vi "test_ReentrantMeasurement_MultipleMeasureCalls_ExecuteInParallel.vi"(8 "error in":errorcluster) -> (0 "error out":errorcluster, 2 "result":string, 3 "pass":bool)   [LabVIEW 2021, in "MeasurementServerTests.lvlib" / "Measurement Service Tests.lvlib"]
uses:
  Measurement Service Tests.lvlib
  Runtime/Measurements/Helpers/TypeDefs/Measurement Server User Settings.ctl
  Runtime/Measurements/Helpers/TypeDefs/Stop Server User Event.ctl
  Runtime/Measurements/Helpers/TypeDefs/Measurement Service Version.ctl
  Continuous Counting Client/controls/Measurement Configuration.ctl
  f8b4024b-4f22-4a1f-8b12-3de1cba605e1.vi
  Runtime/Measurements/NI Measurement Plug-In SDK.lvlib
  Continuous Counting Client/Continuous Counting Client.lvlib
  Continuous Counting Measurement/Continuous Counting Measurement.lvclass
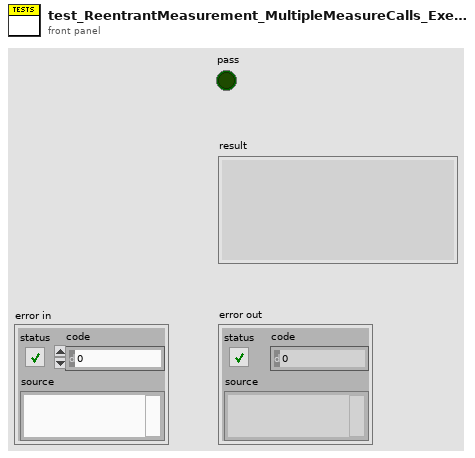
[diagram p1: front panel]
types:
  T1 = typedef "MeasurementServerTests.lvlib/Measurement Service Tests.lvlib/Continuous Counting Client.lvlib/Measurement Configuration.ctl" = cluster{"ms update interval":u32}
  T2 = typedef "NI Measurement Plug-In SDK.lvlib/Measurement Service Version.ctl" = enum16{"V1", "V2"}
  T3 = typedef "NI Measurement Plug-In SDK.lvlib/Measurement Server User Settings.ctl" = cluster{"stop server":T4, "measurement service versions":T2[]}
  T4 = typedef "NI Measurement Plug-In SDK.lvlib/Stop Server User Event.ctl" = refnum<user-event>
  T5 = typedef "grpc-lvsupport-release.lvlib/grpcId.ctl" = u64
  T6 = typedef "MeasurementServerTests.lvlib/Measurement Service Tests.lvlib/Continuous Counting Client.lvlib/Measurement Results.ctl" = cluster{"current count":i64}
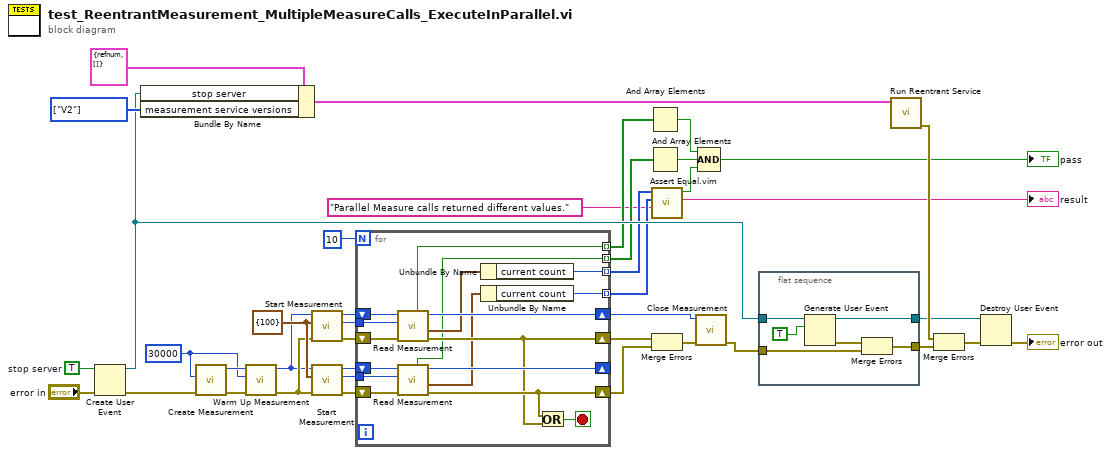
[diagram p0: block diagram]
diagram:
  w5 = 30000 ("ms timeout")
  w35 = T1 {"ms update interval"=100} ("measurement configuration")
  w38 = TRUE  # stop server
  w39 = T2[] [enum."V2"] items=["V1", "V2"] ("measurement service versions")
  n1 = Create User Event(user event datatype=w38, error in="error in") -> (user event=w22:refnum<user-event>, error out=w23:errorcluster)
  n2 = Bundle By Name(cluster=T3 {"stop server"=refnum, "measurement service versions"=[]} ("server settings"), "stop server"=w22, "measurement service versions"=w39) -> (w37:T3)
  n3 = call "Create Measurement.vi"("error in"=w23, "ms timeout"=w5) -> ("error out"=w9:errorcluster, "gRPCid out"=w7:T5)  [unwired: 8 in]
  n4 = call "Warm Up Measurement.vi"("error in"=w9, "timeout (ms)"=w5, "gRPC ID"=w7) -> ("error out"=w8:errorcluster, "gRPC ID out"=w6:T5)  [unwired: 6 in, 1 out]
  n5 = call "Start Measurement.vi"("error in"=w8, "measurement configuration"=w35, "gRPCid in"=w6) -> ("error out"=w32:errorcluster, "call id"=w33:T5, "gRPCid out"=w34:T5)  [unwired: 6 in]
  n6 = call "Start Measurement.vi"("error in"=w8, "measurement configuration"=w35, "gRPCid in"=w6) -> ("error out"=w30:errorcluster, "call id"=w29:T5, "gRPCid out"=w31:T5)  [unwired: 6 in]
  n7 = for {
    N: 10 -> [_]
    tunnel: w33 -> [w56]
    tunnel: w29 -> [w52]
    shift-right: [w51] -> w27
    shift-left: w34 -> [w57]
    shift-right: [w45] -> w25
    shift-left: w32 -> [w55]
    shift-right: [w50] -> _
    shift-left: w31 -> [w54]
    shift-right: [w46] -> w26
    shift-left: w30 -> [w53]
    tunnel: [w42] -> w19 mode=indexing
    tunnel: [w44] -> w20 mode=indexing
    tunnel: [w49] -> w18 mode=indexing
    tunnel: [w48] -> w17 mode=indexing
    stop <- w47 stop-if-true
    n8 = call "Read Measurement.vi"("error in"=w55, "call id in"=w56, "gRPCid in"=w57) -> ("error out"=w45:errorcluster, "measurement results"=w43:T6, "gRPCid out"=w51:T5, "measure success?"=w44:bool)  [unwired: 4 in, 1 out]
    n9 = call "Read Measurement.vi"("error in"=w53, "call id in"=w52, "gRPCid in"=w54) -> ("error out"=w46:errorcluster, "measurement results"=w41:T6, "gRPCid out"=w50:T5, "measure success?"=w42:bool)  [unwired: 4 in, 1 out]
    n10 = Unbundle By Name(w43) -> ("current count"=w49:i64)
    n11 = Unbundle By Name(w41) -> ("current count"=w48:i64)
    n12 = Or(x=w46, y=w45) -> (x .or. y?=w47:bool)
  }
  n13 = And Array Elements(Boolean array=w20) -> (logical AND=w14:bool)
  n14 = And Array Elements(Boolean array=w19) -> (logical AND=w13:bool)
  n15 = call "Assert Equal.vim"("failure message"="Parallel Measure calls returned different values.", "actual value"=w17, "expected value"=w18) -> ("message"=→"result":string, "equal?"=w15:bool)  [unwired: 7 in]
  n16 = Merge Errors(w25, w26) -> (w24:errorcluster)
  n17 = call "Close Measurement.vi"("error in"=w24, "gRPCid in"=w27) -> ("error out"=w10:errorcluster)  [unwired: 9 in]
  n18 = Compound Arithmetic op=AND(w14, w13, w15) -> (→"pass":bool)
  n19 = flat-sequence {
    tunnel: w22 -> [w62]
    tunnel: [w61] -> w1
    tunnel: [w60] -> w4
    tunnel: w10 -> [w59]
    frame #0 {
      n20 = Generate User Event(user event=w62, event data cluster=TRUE ("event data")) -> (user event out=w61:refnum<user-event>, error out=w63:errorcluster)  [unwired: 2 in]
      n21 = Merge Errors(w63, w59) -> (w60:errorcluster)
    }
  }
  n22 = call "Run Reentrant Service.vi"("server settings"=w37) -> ("error out"=w21:errorcluster)  [unwired: 10 in]
  n23 = Merge Errors(w21, w4) -> (w3:errorcluster)
  n24 = Destroy User Event(user event=w1, error in=w3) -> (error out=→"error out":errorcluster)
